vi "GetDefaultXhairs.vi"(0 "appended array 2":string[](array[string])) -> (1 "appended array":string[](array[string]), 2 "appended array 4":string[](array[string]), 3 "appended array 6":string[](array[string]), 4 "appended array 8":string[](array[string]))   [LabVIEW 2013]
uses:
  Shared/MySQL/Preset Query Enum.ctl
panel:
  out "subarray 4":string[](array[string])
  out "element 16":string
  out "element 15":string
  out "element 14":string
  out "element 13":string
  out "subarray 3":string[](array[string])
  out "element 12":string
  out "element 11":string
  out "element 10":string
  out "element 9":string
  out "subarray 2":string[](array[string])
  out "element 8":string
  out "element 7":string
  out "element 6":string
  out "element 5":string
  out "subarray":string[](array[string])
  out "element 4":string
  out "element 3":string
  out "element":string
  out "element 2":string
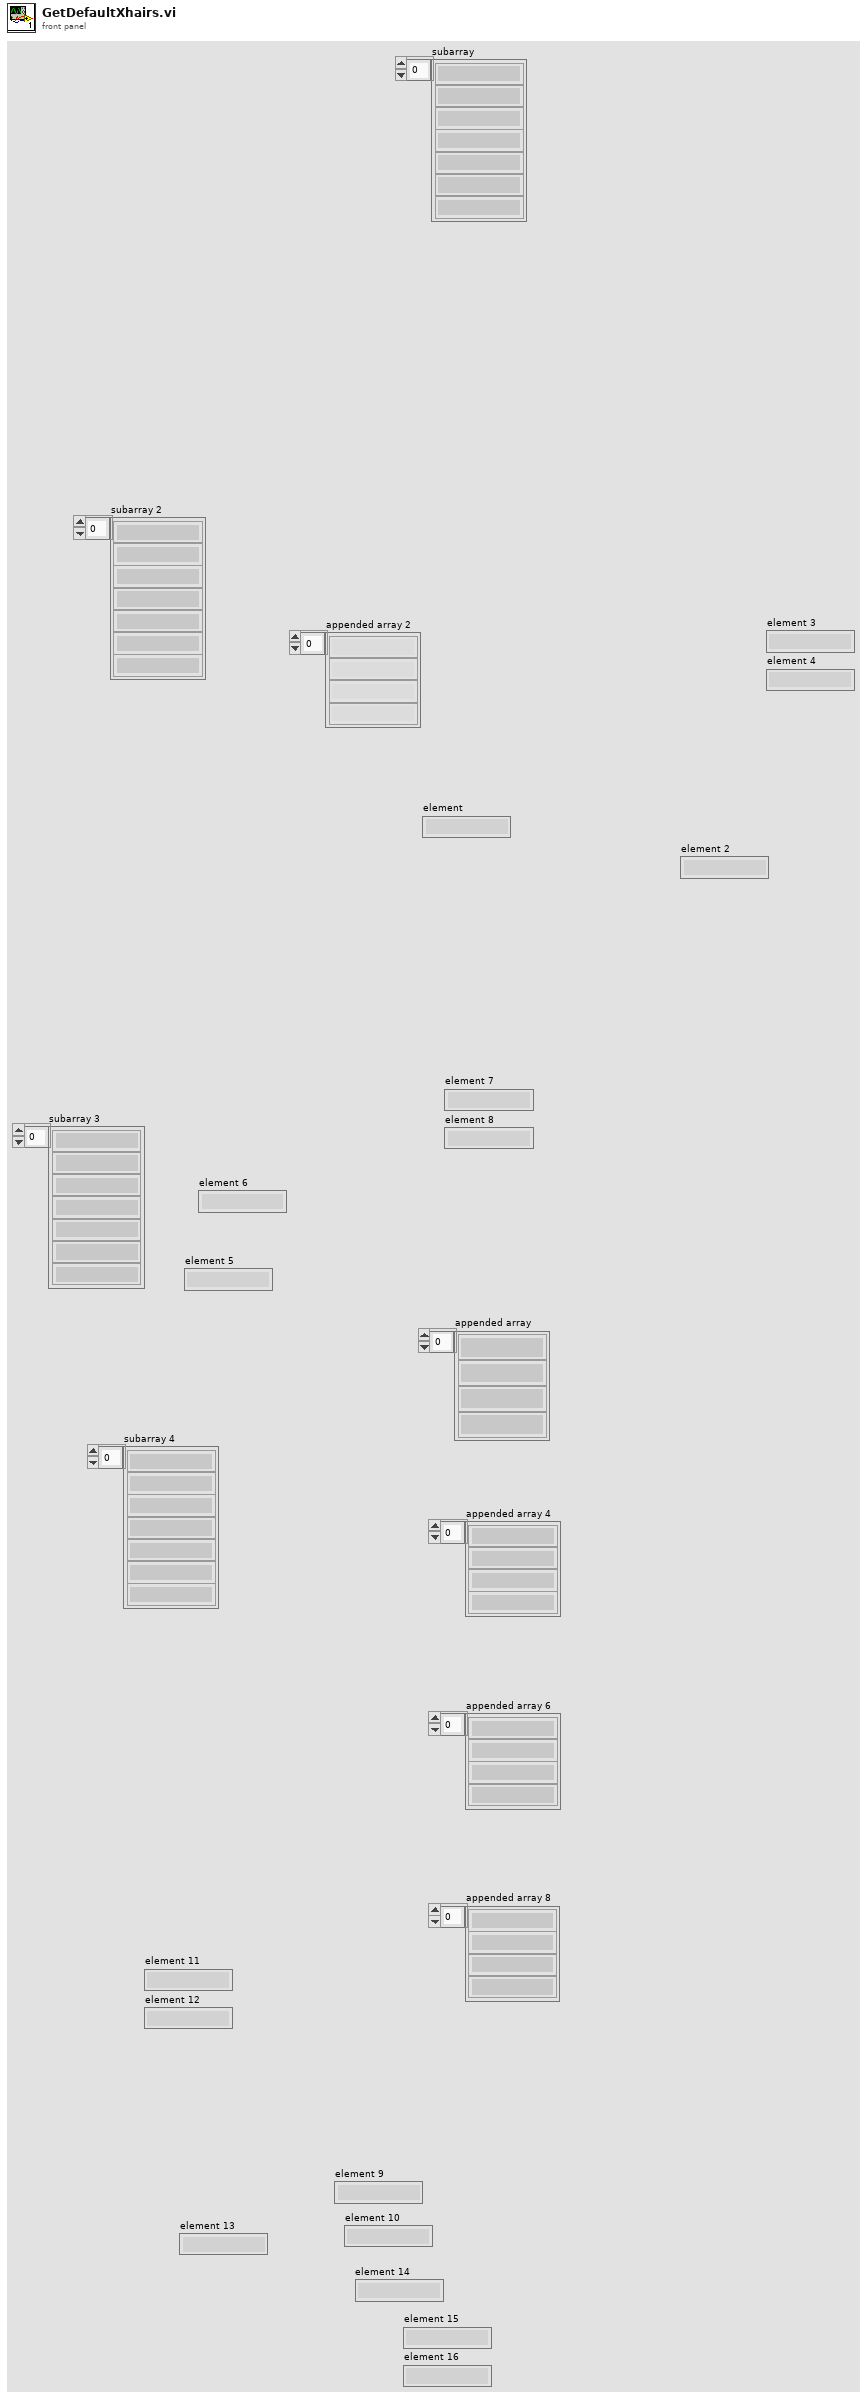
[diagram p1: front panel]
types:
  T1 = typedef "Preset Query Enum.ctl" = enum16{"Get Locations", "Get all IPs and MACs", "Get classes", "Get expt variables to set at scanstart for particular device", "Get expt devices and variables with start values", "Get expt devices and variables (with data to get)", "Get expt devices with data to get", "Get Expt devices and GUIs", "Get all devices basic properties", "Get Virtual Devices Core Info", "Get Expt names", "Get experiment basic properties", "Get experiment alarm variables", "Get MC Ports", "Get device network comm port", "Get devicetype lvclass path", "Get basic device properties", "Get Init Order", "Get all setable variables of a device", "Get device variable aliases", "Get force values of all settable variables", "Get all variables of a devicetype", "Get all variables of a device", "Get plotter details", "Get Saved Scans", "Get Scan Info", "GetGeneralGUIs", "Get expt for plotter", "Get plotter IDs from expt", "Get all devices", "Get all Virtual Devices", "Get all aliases", "Get variable and device info for Virtual Device", "GetItemLocatorIP", "Get IPs for GUIs", "Get DeviceType from Device", "GetLocalPortRange", "GetDevicePresetVariables", "Get Device Configuration", "GetAllPresetNames", "GetAllConfigurationNames", "GetPresetDeviceNames"}
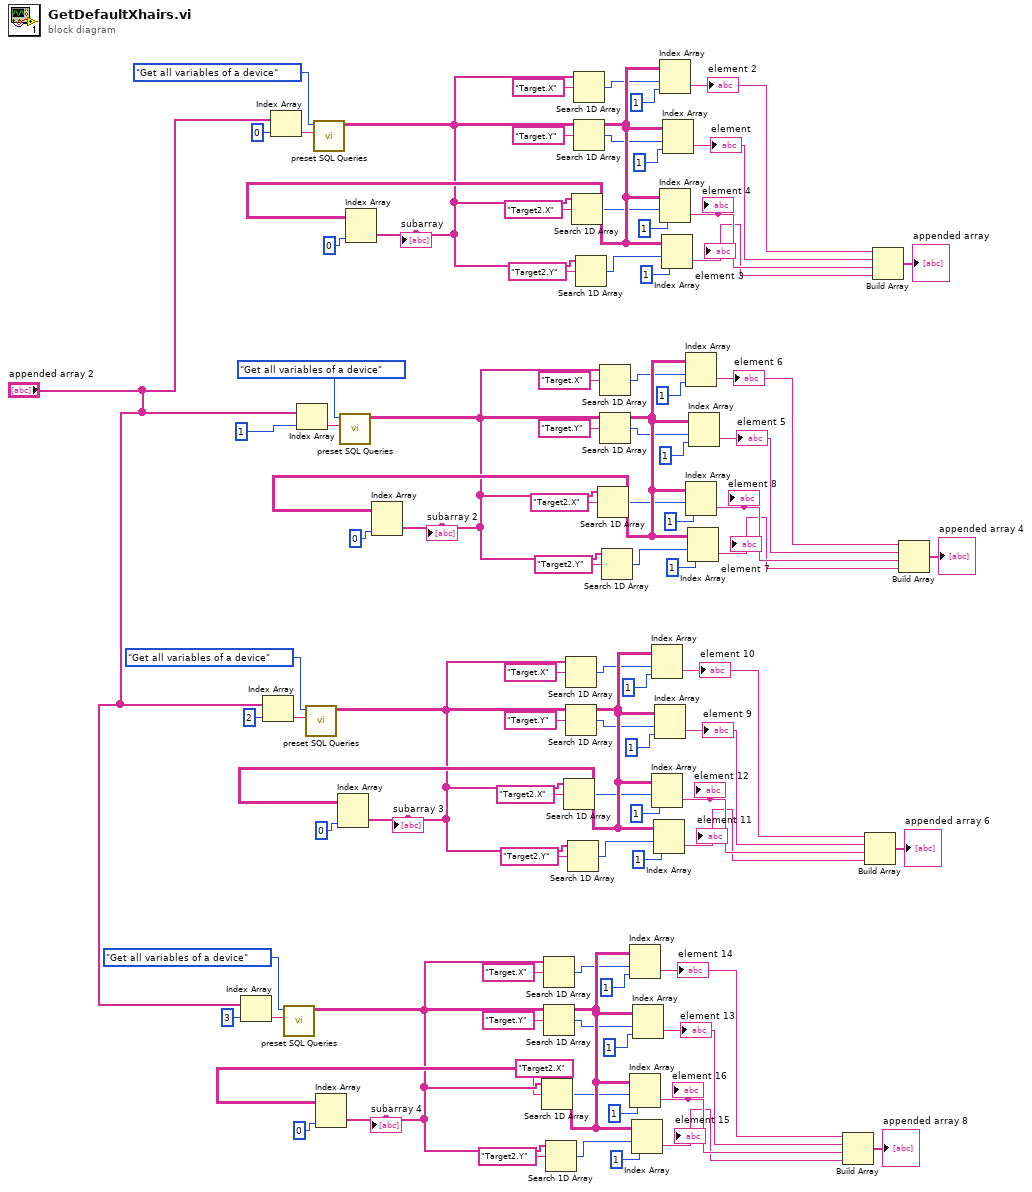
[diagram p0: block diagram]
diagram:
  n1 = Index Array(array="appended array 2", index=3) -> (element=w20:string)
  n2 = Index Array(array="appended array 2", index=2) -> (element=w43:string)
  n3 = Index Array(array="appended array 2", index=0) -> (element=w89:string)
  n4 = call "preset SQL Queries.vi"("Device/Devicetype name\n/Plotter.id/ScanName#"=w20, "Preset Query"=Preset_Query_Enum."Get all variables of a device") -> ("data"=w11:string[][])  [unwired: 7 in, 2 out]
  n5 = Index Array(array="appended array 2", index=1) -> (element=w66:string)
  n6 = call "preset SQL Queries.vi"("Device/Devicetype name\n/Plotter.id/ScanName#"=w43, "Preset Query"=Preset_Query_Enum."Get all variables of a device") -> ("data"=w34:string[][])  [unwired: 7 in, 2 out]
  n7 = call "preset SQL Queries.vi"("Device/Devicetype name\n/Plotter.id/ScanName#"=w89, "Preset Query"=Preset_Query_Enum."Get all variables of a device") -> ("data"=w80:string[][])  [unwired: 7 in, 2 out]
  n8 = Index Array(array=w11, index (col)=0 ("disabled index (col)")) -> (element=w6:string[])  [unwired: 1 in]
  "subarray 4" <- w6
  n9 = Index Array(array=w34, index (col)=0 ("disabled index (col)")) -> (element=w29:string[])  [unwired: 1 in]
  "subarray 3" <- w29
  n10 = call "preset SQL Queries.vi"("Device/Devicetype name\n/Plotter.id/ScanName#"=w66, "Preset Query"=Preset_Query_Enum."Get all variables of a device") -> ("data"=w57:string[][])  [unwired: 7 in, 2 out]
  n11 = Index Array(array=w80, index (col)=0 ("disabled index (col)")) -> (element=w75:string[])  [unwired: 1 in]
  "subarray" <- w75
  n12 = Index Array(array=w57, index (col)=0 ("disabled index (col)")) -> (element=w52:string[])  [unwired: 1 in]
  "subarray 2" <- w52
  n13 = Search 1D Array(1D array=w6, element="Target2.X") -> (index of element=w3:i32)  [unwired: 1 in]
  n14 = Search 1D Array(1D array=w6, element="Target.X") -> (index of element=w9:i32)  [unwired: 1 in]
  n15 = Search 1D Array(1D array=w6, element="Target.Y") -> (index of element=w7:i32)  [unwired: 1 in]
  n16 = Search 1D Array(1D array=w6, element="Target2.Y") -> (index of element=w2:i32)  [unwired: 1 in]
  n17 = Search 1D Array(1D array=w29, element="Target2.X") -> (index of element=w26:i32)  [unwired: 1 in]
  n18 = Search 1D Array(1D array=w29, element="Target.X") -> (index of element=w32:i32)  [unwired: 1 in]
  n19 = Search 1D Array(1D array=w29, element="Target.Y") -> (index of element=w30:i32)  [unwired: 1 in]
  n20 = Search 1D Array(1D array=w29, element="Target2.Y") -> (index of element=w25:i32)  [unwired: 1 in]
  n21 = Search 1D Array(1D array=w75, element="Target2.X") -> (index of element=w72:i32)  [unwired: 1 in]
  n22 = Search 1D Array(1D array=w75, element="Target.X") -> (index of element=w78:i32)  [unwired: 1 in]
  n23 = Search 1D Array(1D array=w75, element="Target.Y") -> (index of element=w76:i32)  [unwired: 1 in]
  n24 = Search 1D Array(1D array=w75, element="Target2.Y") -> (index of element=w71:i32)  [unwired: 1 in]
  n25 = Search 1D Array(1D array=w52, element="Target2.X") -> (index of element=w49:i32)  [unwired: 1 in]
  n26 = Search 1D Array(1D array=w52, element="Target.X") -> (index of element=w55:i32)  [unwired: 1 in]
  n27 = Search 1D Array(1D array=w52, element="Target.Y") -> (index of element=w53:i32)  [unwired: 1 in]
  n28 = Search 1D Array(1D array=w52, element="Target2.Y") -> (index of element=w48:i32)  [unwired: 1 in]
  n29 = Index Array(array=w11, index (row)=w9, index (col)=1 ("disabled index (col)")) -> (element=w17:string)
  "element 14" <- w17
  n30 = Index Array(array=w11, index (row)=w3, index (col)=1 ("disabled index (col)")) -> (element=w15:string)
  "element 16" <- w15
  n31 = Index Array(array=w11, index (row)=w2, index (col)=1 ("disabled index (col)")) -> (element=w14:string)
  "element 15" <- w14
  n32 = Index Array(array=w11, index (row)=w7, index (col)=1 ("disabled index (col)")) -> (element=w16:string)
  "element 13" <- w16
  n33 = Index Array(array=w34, index (row)=w32, index (col)=1 ("disabled index (col)")) -> (element=w40:string)
  "element 10" <- w40
  n34 = Index Array(array=w34, index (row)=w26, index (col)=1 ("disabled index (col)")) -> (element=w38:string)
  "element 12" <- w38
  n35 = Index Array(array=w34, index (row)=w25, index (col)=1 ("disabled index (col)")) -> (element=w37:string)
  "element 11" <- w37
  n36 = Index Array(array=w34, index (row)=w30, index (col)=1 ("disabled index (col)")) -> (element=w39:string)
  "element 9" <- w39
  n37 = Index Array(array=w80, index (row)=w78, index (col)=1 ("disabled index (col)")) -> (element=w86:string)
  "element 2" <- w86
  n38 = Index Array(array=w80, index (row)=w72, index (col)=1 ("disabled index (col)")) -> (element=w84:string)
  "element 4" <- w84
  n39 = Index Array(array=w80, index (row)=w71, index (col)=1 ("disabled index (col)")) -> (element=w83:string)
  "element 3" <- w83
  n40 = Index Array(array=w80, index (row)=w76, index (col)=1 ("disabled index (col)")) -> (element=w85:string)
  "element" <- w85
  n41 = Index Array(array=w57, index (row)=w55, index (col)=1 ("disabled index (col)")) -> (element=w63:string)
  "element 6" <- w63
  n42 = Index Array(array=w57, index (row)=w49, index (col)=1 ("disabled index (col)")) -> (element=w61:string)
  "element 8" <- w61
  n43 = Index Array(array=w57, index (row)=w48, index (col)=1 ("disabled index (col)")) -> (element=w60:string)
  "element 7" <- w60
  n44 = Index Array(array=w57, index (row)=w53, index (col)=1 ("disabled index (col)")) -> (element=w62:string)
  "element 5" <- w62
  n45 = Build Array(w17, w16, w15, w14) -> (→"appended array 8":string[])
  n46 = Build Array(w40, w39, w38, w37) -> (→"appended array 6":string[])
  n47 = Build Array(w86, w85, w84, w83) -> (→"appended array":string[])
  n48 = Build Array(w63, w62, w61, w60) -> (→"appended array 4":string[])
